vi "Finalizing Turn.vi"(7 "Actor in":refnum<class "Actor.lvclass">, 8 "Error in":errorcluster) -> (0 "Error out":errorcluster, 2 "Proceed To Tearing Down":bool, 5 "Actor out":refnum<class "Actor.lvclass">)   [LabVIEW 2020, in "jettl.lvlib"]
uses:
  jettl.lvlib
  Lifetime.ctl
  Actor Specific/Actor Specific.lvlib
  Actor/Actor.lvclass
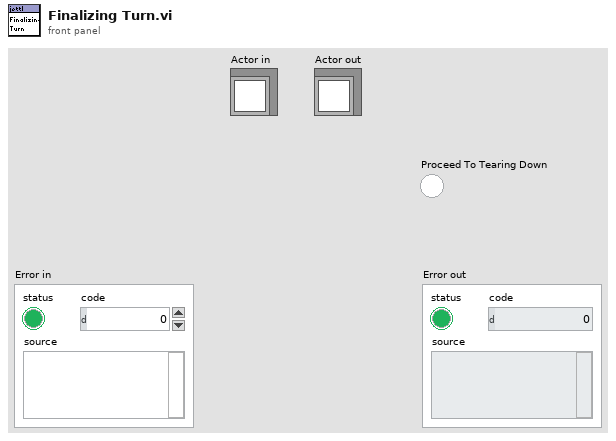
[diagram p1: front panel]
types:
  T1 = typedef "jettl.lvlib/Lifetime.ctl" = enum16{"Init", "Spawn", "Setup", "Teardown Before Running", "Running", "Stop Called", "Stopping With Children", "Stopping Without Children", "Teardown After Running", "Stopped"}
  T2 = typedef "jettl.lvlib/Child Aliases.ctl" = set{string}
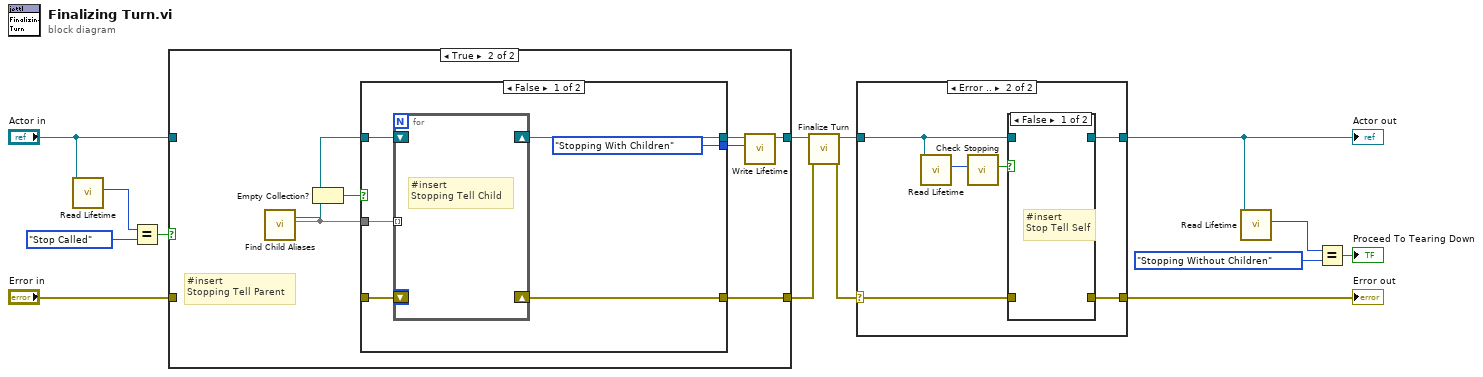
[diagram p0: block diagram]
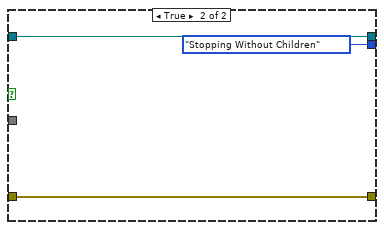
[diagram p3: hidden frame]
diagram:
  n1 = call-dynamic "Read Lifetime.vi"("Actor in"="Actor in") -> ("Lifetime"=w3:T1)  [unwired: 10 in]
  n2 = Equal?(x=w3, y=Lifetime."Stop Called") -> (x = y?=w8:bool)
  n3 = case shown="True" w8 {
    tunnel: "Error in" -> [w16 w23]
    tunnel: [w16 w26] -> w6
    tunnel: [w15 w20] -> w5
    tunnel: "Actor in" -> [w15 w24]
    frame False {
    }
    frame True {
      # "#insert\nStopping Tell Parent"
      n4 = call "Find Child Aliases.vi"("Actor in"=w18) -> ("Child Aliases"=w17:T2)  [unwired: 10 in]
      n5 = Empty Collection?(1:w17) -> (0:w25:bool)
      n6 = case shown="False" w25 {
        tunnel: [w32 w37] -> w22
        tunnel: [w31 w37] -> w26
        tunnel: [Lifetime."Stopping With Children" ("Lifetime") Lifetime."Stopping Without Children" ("Lifetime")] -> w19
        tunnel: [w30 w38] -> w18
        tunnel: [w29 w38] -> w21
        tunnel: w17 -> [w28 _]
        frame False {
          n7 = for {
            tunnel: w28 -> [w33] mode=indexing
            shift-right: [w35] -> w31
            shift-left: w32 -> [w36]
            shift-right: [w34] -> w29
            shift-left: w30 -> [_]
            # "#insert\nStopping Tell Child"
          }
        }
        frame True {
        }
      }
      n8 = call-dynamic "Write Lifetime.vi"("Lifetime"=w19, "Actor in"=w21) -> ("Actor out"=w20:refnum<class "Actor.lvclass">)  [unwired: 9 in]
    }
  }
  n9 = call-dynamic "Finalize Turn.vi"("Error in"=w6, "Actor in"=w5) -> ("Error out"=w12:errorcluster, "Actor out"=w11:refnum<class "Actor.lvclass">)  [unwired: 8 in]
  n10 = case shown="Error .." w12 {
    selector: w12 -> [_ w44]
    tunnel: [w40 w46] -> w2
    tunnel: [_ w45] -> w10
    tunnel: w11 -> [w40 w42]
    frame No Error {
    }
    frame Error {
      n11 = call-dynamic "Read Lifetime.vi"("Actor in"=w42) -> ("Lifetime"=w41:T1)  [unwired: 10 in]
      n12 = call "Check Stopping.vi"("Lifetime"=w41) -> ("Stopping"=w43:bool)  [unwired: 10 in]
      n13 = case shown="False" w43 {
        tunnel: [w47 w50] -> w46
        tunnel: w42 -> [w48 w50]
        tunnel: w44 -> [_ w49]
        tunnel: [_ w49] -> w45
        frame False {
          # "#insert\nStop Tell Self"
        }
        frame True {
        }
      }
    }
  }
  "Actor out" <- w2
  "Error out" <- w10
  n14 = call-dynamic "Read Lifetime.vi"("Actor in"=w2) -> ("Lifetime"=w1:T1)  [unwired: 10 in]
  n15 = Equal?(x=w1, y=Lifetime."Stopping Without Children") -> (x = y?=→"Proceed To Tearing Down":bool)
